vi "Start Compile.vi"(11 "FPGAtarget in":refnum<class "FPGATarget.lvclass">) -> (3 "FPGAtarget out":refnum<class "FPGATarget.lvclass">)   [LabVIEW 2020, in "NI_TargetHelper.lvlib" / "FPGATarget.lvclass"]
uses:
  <vilib>/TargetSupport/NI_TargetHelper/FPGATarget/FPGATarget.lvclass
  <vilib>/TargetSupport/NI_TargetHelper/FPGATarget/FPGATarget.lvclass/FPGATarget.ctl
  <vilib>/TargetSupport/NI_TargetHelper/NI_TargetHelper.lvlib
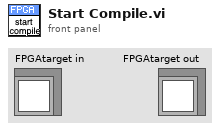
[diagram p1: front panel]
types:
  T1 = typedef "NI_TargetHelper.lvlib/Instance VIref.ctl" = refnum<vi>
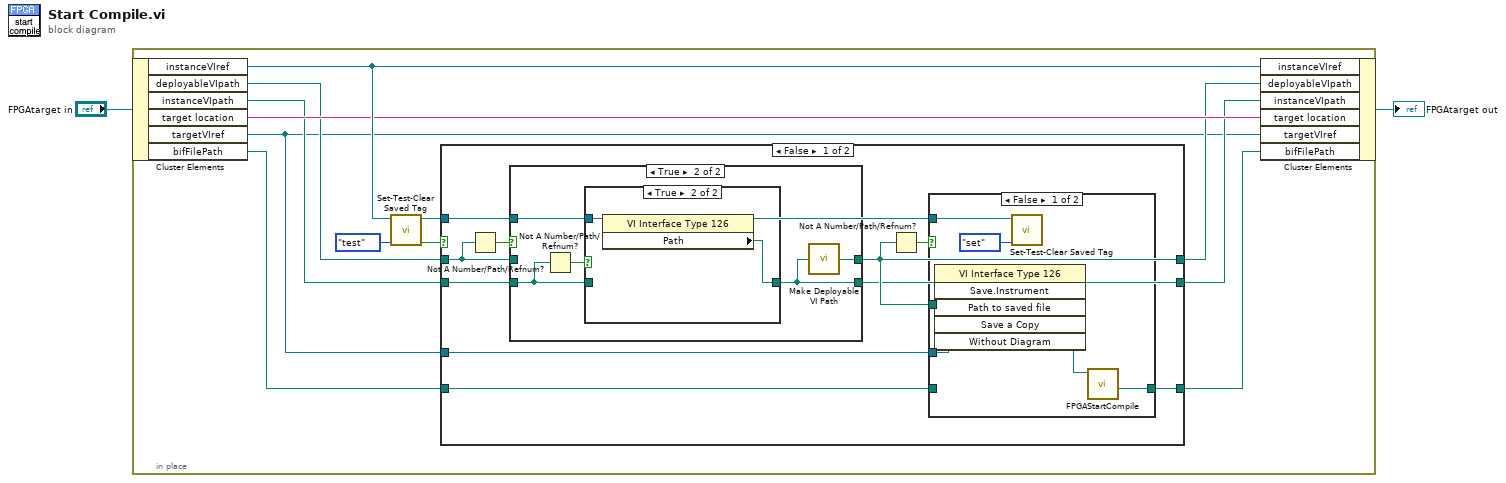
[diagram p0: block diagram]
diagram:
  n1 = in-place {
    n2 = in-place-cluster #1("FPGAtarget in") -> ("instanceVIref"=w14:T1, "deployableVIpath"=w9:path, "instanceVIpath"=w7:path, "target location"=w10:string, "targetVIref"=w5:T1, "bifFilePath"=w3:path)
    n3 = call <vilib>:"Set-Test-Clear Saved Tag.vi"("op"=enum16{"test", "clear", "set"}."test", "instVIref"=w14) -> ("saved"=w11:bool, "instVIref out"=w13:T1)  [unwired: 8 in]
    n4 = case shown="False" w11 {
      tunnel: w13 -> [w19 _]
      tunnel: w5 -> [w17 _]
      tunnel: w7 -> [w23 w43]
      tunnel: w9 -> [w22 w44]
      tunnel: [w20 w44] -> w8
      tunnel: [w18 w43] -> w6
      tunnel: [w16 w42] -> w4
      tunnel: w3 -> [w15 w42]
      frame False {
        n5 = Not A Number/Path/Refnum?(number/path/refnum=w22) -> (NaN/Path/Refnum?=w24:bool)
        n6 = case shown="True" w24 {
          tunnel: w23 -> [w32 w35]
          tunnel: w22 -> [w33 _]
          tunnel: [w33 w38] -> w20
          tunnel: w19 -> [_ w36]
          tunnel: [w32 w34] -> w18
          frame False {
          }
          frame True {
            n7 = Not A Number/Path/Refnum?(number/path/refnum=w35) -> (NaN/Path/Refnum?=w37:bool)
            n8 = case shown="True" w37 {
              tunnel: w36 -> [_ w41]
              tunnel: [w39 w40] -> w34
              tunnel: w35 -> [w39 _]
              frame False {
              }
              frame True {
                n9 = property class="VI Interface Type 126"(reference=w41) -> ("Path"=w40:path)  [unwired: 1 in, 2 out]
              }
            }
            n10 = call <vilib>:"Make Deployable VI Path.vi"("instance path"=w34) -> ("deployable path"=w38:path)
          }
        }
        n11 = Not A Number/Path/Refnum?(number/path/refnum=w20) -> (NaN/Path/Refnum?=w21:bool)
        n12 = case shown="False" w21 {
          tunnel: w17 -> [w30 _]
          tunnel: w20 -> [w29 _]
          tunnel: w19 -> [w27 _]
          tunnel: [w25 w31] -> w16
          tunnel: w15 -> [_ w31]
          frame False {
            n13 = invoke class="VI Interface Type 126" method="Save.Instrument"(reference=w30, "Path to saved file"=w29) -> (reference out=w26:T1)  [unwired: 4 in, 5 out]
            n14 = call <vilib>:"Set-Test-Clear Saved Tag.vi"("op"=enum16{"test", "clear", "set"}."set", "instVIref"=w27) -> ()  [unwired: 8 in, 2 out]
            n15 = call <vilib>:"FPGAStartCompile.vi"("viref"=w26) -> ("bitfile path when compile done"=w25:path)  [unwired: 10 in]
          }
          frame True {
          }
        }
      }
      frame True {
      }
    }
    n16 = in-place-cluster #1("instanceVIref"=w14, "deployableVIpath"=w8, "instanceVIpath"=w6, "target location"=w10, "targetVIref"=w5, "bifFilePath"=w4) -> (→"FPGAtarget out":refnum<class "FPGATarget.lvclass">)
  }
